vi "serial test.vi"() -> ()   [LabVIEW 2016, in "navX Library.lvlib"]
uses:
  navX Library.lvlib
panel:
  in  "write data":string
  in  "port":string="/dev/ttyACM0"
  out "serial read return value":i32
  out "read data":string
  out "serial write return value":i32
  out "portHandle out":i32
  out "error out":errorcluster
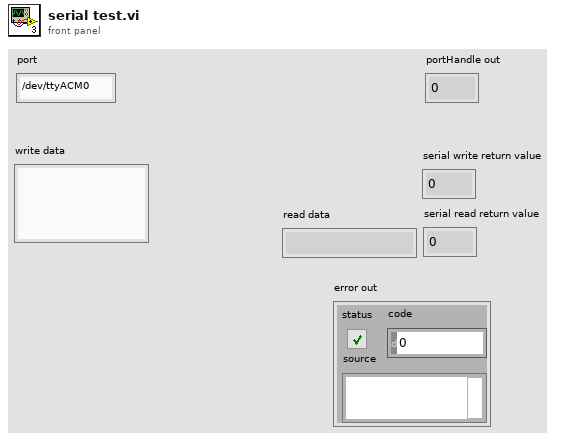
[diagram p1: front panel]
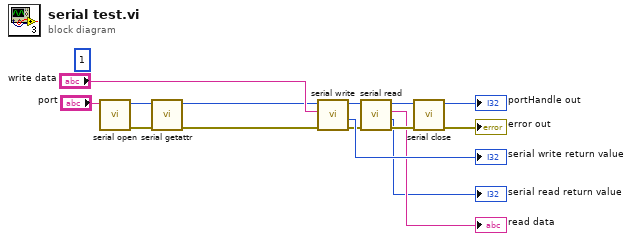
[diagram p0: block diagram]
diagram:
  (unwired) 1 ("cnt")
  n1 = call "serial open.vi"("port"="port") -> ("error out"=w2:errorcluster, "portHandle"=w4:i32)  [unwired: 9 in]
  n2 = call "serial getattr.vi"("error in (no error)"=w2, "portHandle in"=w4) -> ("error out"=w1:errorcluster, "portHandle out"=w3:i32)  [unwired: 7 in, 1 out]
  n3 = call "serial write.vi"("error in (no error)"=w1, "data"="write data", "portHandle in"=w3) -> ("error out"=w8:errorcluster, "return value"=→"serial write return value":i32, "portHandle out"=w10:i32)  [unwired: 6 in]
  n4 = call "serial read.vi"("error in (no error)"=w8, "portHandle in"=w10) -> ("error out"=w7:errorcluster, "return value"=→"serial read return value":i32, "data"=→"read data":string, "portHandle out"=w9:i32)  [unwired: 6 in]
  n5 = call "serial close.vi"("error in (no error)"=w7, "portHandle in"=w9) -> ("error out"=→"error out":errorcluster, "portHandle out"=→"portHandle out":i32)  [unwired: 8 in]
